vi "mqttConfigStore.vi"(0 "mqtt.lvclass in":refnum<class "mqtt.lvclass">, 2 "function":T1=enum."set", 11 "error in (no error)":errorcluster) -> (4 "mqtt.lvclass out":refnum<class "mqtt.lvclass">, 15 "error out":errorcluster)   [LabVIEW 2019, in "mqtt.lvclass"]
uses:
  mqtt.lvclass
  mqttConfigFunction.ctl
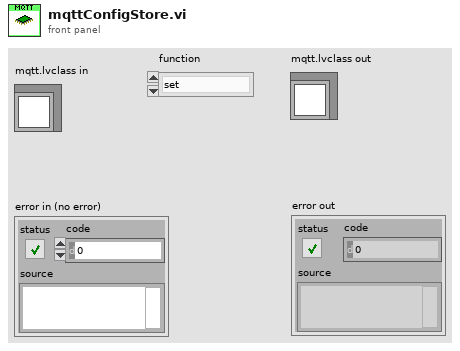
[diagram p1: front panel]
types:
  T1 = typedef "mqtt.lvclass/mqttConfigFunction.ctl" = enum16{"init", "deinit", "set", "get"}
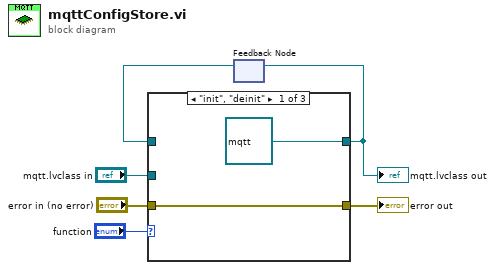
[diagram p0: block diagram]
diagram:
  n1 = feedback #1() -> (w4:refnum<class "mqtt.lvclass">)  [unwired: 1 in]
  n2 = case shown="\"init\", \"deinit\"" "function" {
    tunnel: [refnum<class "mqtt.lvclass"> refnum ("mqtt.lvclass") w9 w11] -> w5
    tunnel: w4 -> [_ _ w11]
    tunnel: "error in (no error)" -> [w7 w10 w12]
    tunnel: [w7 w10 w12] -> w2
    tunnel: "mqtt.lvclass in" -> [_ w9 _]
    frame "init", "deinit" {
    }
    frame "set" {
    }
    frame "get" {
    }
  }
  "error out" <- w2
  "mqtt.lvclass out" <- w5
  n3 = feedback-in #1(w5) -> ()
